vi "Generate inverse weighted window.vi"(11 "Window size":i32=500) -> (1 "sum":dbl, 3 "Waveform Graph":dbl[](graph))   [LabVIEW 2013]
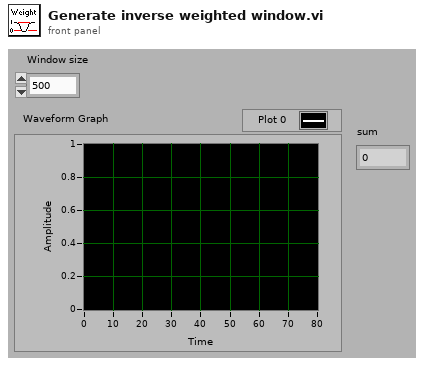
[diagram p1: front panel]
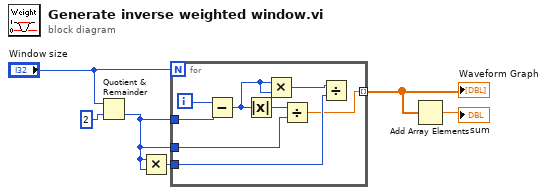
[diagram p0: block diagram]
diagram:
  n1 = Quotient & Remainder(x="Window size", y=2) -> (floor(x/y)=w4:i32)  [unwired: 1 out]
  n2 = Multiply(x=w4, y=w4) -> (x*y=w3:i32)
  n3 = for {
    N: "Window size" -> [_]
    tunnel: [w7] -> w2 mode=indexing
    tunnel: w4 -> [w13]
    tunnel: w4 -> [w12]
    tunnel: w3 -> [w9]
    i -> [w14]
    n4 = Subtract(x=w14, y=w13) -> (x-y=w11:i32)
    n5 = Absolute Value(x=w11) -> (abs(x)=w8:i32)
    n6 = Multiply(x=w11, y=w11) -> (x*y=w10:i32)
    n7 = Divide(x=w8, y=w12) -> (x/y=w7:dbl)
    n8 = Divide(x=w10, y=w9) -> ()  [unwired: 1 out]
  }
  "Waveform Graph" <- w2
  n9 = Add Array Elements(numeric array=w2) -> (sum=→"sum":dbl)
